vi "Build_ch_list_from_array.vi"(9 "Differential\nMode":bool, 10 "Scan array":bool[][](array[boolean]), 11 "Ch definition path (dialog if empty)":path) -> (2 "number of contacts":i32, 3 "Scan String":string)   [LabVIEW 2013]
panel:
  # "Columns=connector no. starting at 1\nRows=inputs starting at 1"
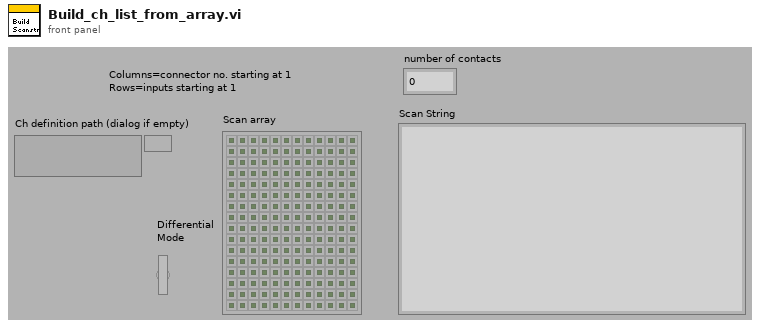
[diagram p1: front panel]
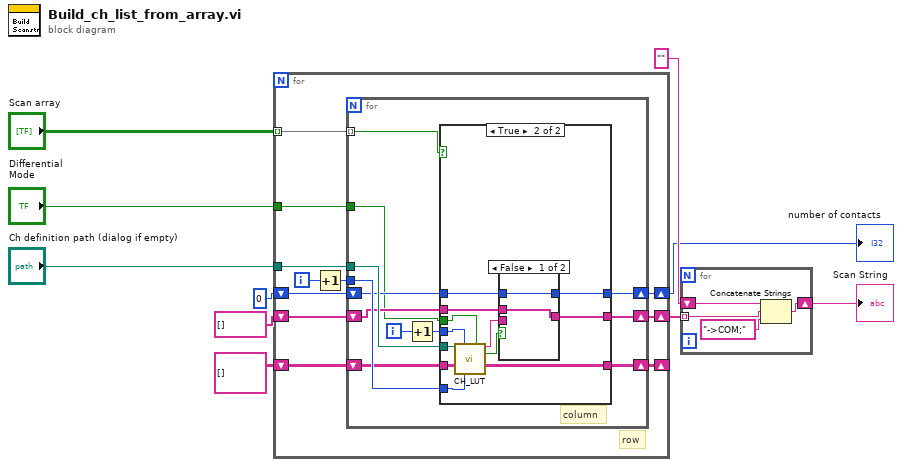
[diagram p0: block diagram]
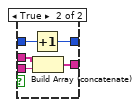
[diagram p3: hidden frame]
diagram:
  n1 = for {
    tunnel: "Scan array" -> [w21] mode=indexing
    tunnel: "Ch definition path (dialog if empty)" -> [w20]
    shift-right: [w17] -> w6
    shift-left: string[] [] -> [w16]
    shift-right: [w15] -> _
    shift-left: string[][] [] ("Channel LUT") -> [w14]
    shift-right: [w12] -> w2
    shift-left: 0 -> [w13]
    tunnel: "Differential\nMode" -> [w11]
    i -> [w19]
    # "row"
    n2 = Increment(x=w19) -> (x+1=w18:i32)
    n3 = for {
      tunnel: w21 -> [w25] mode=indexing
      tunnel: w20 -> [w33]
      tunnel: w18 -> [w31]
      shift-right: [w29] -> w17
      shift-left: w16 -> [w28]
      shift-right: [w27] -> w15
      shift-left: w14 -> [w26]
      shift-right: [w23] -> w12
      shift-left: w13 -> [w24]
      tunnel: w11 -> [w22]
      i -> [w32]
      # "column"
      n4 = Increment(x=w32) -> (x+1=w30:i32)
      n5 = case shown="True" w25 {
        tunnel: w33 -> [_ w48]
        tunnel: w30 -> [_ w41]
        tunnel: w31 -> [_ w40]
        tunnel: [w36 w45] -> w29
        tunnel: w28 -> [w36 w44]
        tunnel: [w35 w43] -> w27
        tunnel: w26 -> [w35 w42]
        tunnel: w24 -> [w34 w39]
        tunnel: [w34 w38] -> w23
        tunnel: w22 -> [_ w37]
        frame False {
        }
        frame True {
          n6 = call "CH_LUT.vi"("file path (dialog if empty)"=w48, "Input#"=w41, "Differential\nMode"=w37, "Channel LUT IN"=w42, "Channel"=w40) -> ("Ch name"=w46:string, "found?"=w47:bool, "Channel LUT"=w43:string[][])  [unwired: 6 in, 2 out]
          n7 = case shown="False" w47 {
            tunnel: w46 -> [_ w55]
            tunnel: [w50 w54] -> w45
            tunnel: w44 -> [w50 w53]
            tunnel: w39 -> [w49 w52]
            tunnel: [w49 w51] -> w38
            frame False {
            }
            frame True {
              n8 = Increment(x=w52) -> (x+1=w51:i32)
              n9 = Build Array (concatenate)(w53, w55) -> (w54:string[])
            }
          }
        }
      }
    }
  }
  "number of contacts" <- w2
  n10 = for {
    tunnel: w6 -> [w59] mode=indexing
    shift-right: [w57] -> w4
    shift-left: "" -> [w56]
    n11 = Concatenate Strings(w56, w59, "->COM;" ("string")) -> (w57:string)
  }
  "Scan String" <- w4
